vi "Home Axis.vi"(8 "error in (no error)":errorcluster, 10 "Axis Name":string, 11 "A3200 in":refnum<class "A3200.lvclass">) -> (0 "error out":errorcluster, 3 "A3200 out":refnum<class "A3200.lvclass">)   [LabVIEW 2016, in "A3200.lvclass"]
uses:
  A3200.lvclass
  A3200.lvclass/A3200.ctl
  Motion.lvclass
  Drivers/Aerotech A3200/Aerotech VIs.lvlib
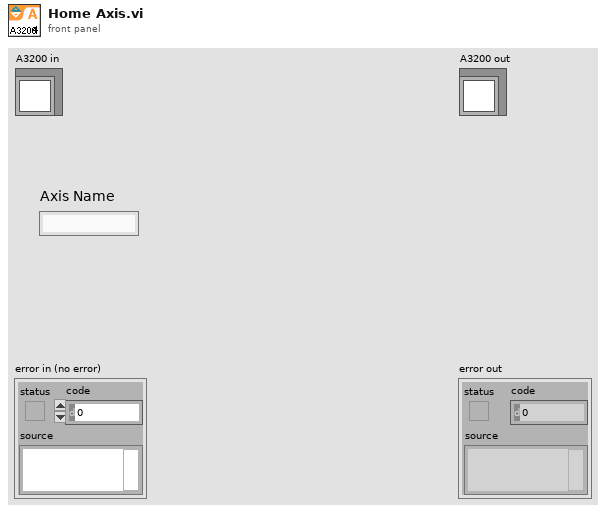
[diagram p1: front panel]
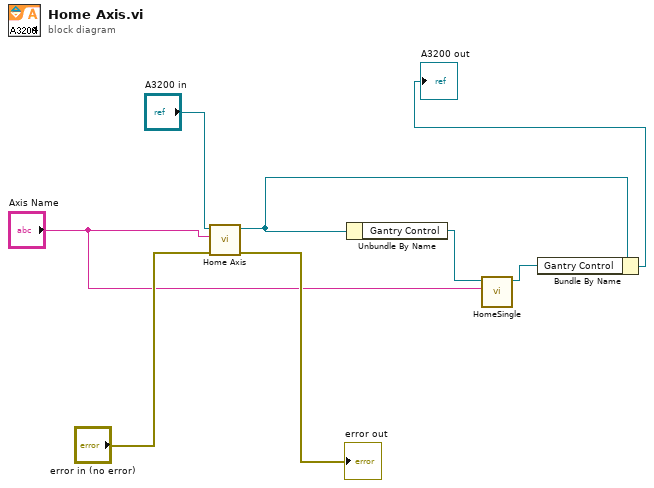
[diagram p0: block diagram]
diagram:
  n1 = call-parent "Home Axis.vi"("error in (no error)"="error in (no error)", "Axis Name"="Axis Name", "Motion in"="A3200 in") -> ("error out"=→"error out":errorcluster, "Motion out"=w2:refnum<class "A3200.lvclass">)  [unwired: 7 in]
  n2 = Unbundle By Name(w2) -> ("Gantry Control"=w5:refnum<k24>)
  n3 = call "HomeSingle.vi"("axis name"="Axis Name", "controller in"=w5) -> ("controller out"=w3:refnum<k24>)  [unwired: 8 in, 1 out]
  n4 = Bundle By Name(cluster=w2, "Gantry Control"=w3) -> (→"A3200 out":refnum<class "A3200.lvclass">)
